vi "InitCamera.vi"(3 "error in":errorcluster, 5 "Scan.lvclass":refnum<class "Scan.lvclass">) -> (0 "error out":errorcluster, 2 "Initialized Camera":T2)   [LabVIEW 2017]
doc: "Creates, and edits acquisitions using the NI Vision Acquisition Express VI.\n\nThe NI Vision Acquisition Wizard is launched by placing the Express VI on the block diagram. Select an acquisition source and configure an acquisition using NI-IMAQ, NI-IMAQdx, or simulate an acquisition by reading an AVI or image files from a folder. After an acquisition is configured, select controls and indicators to be able to programmatically set in LabVIEW. Double-click the Vision Acquisition Express VI to edit the acquisition.\n\nNote: Any images created by the Express VI need to be disposed after use. Use the IMAQ Dispose.vi to cleanup the images output by the Express VI when they are no longer needed."
uses:
  classes/Scans/Scan.lvclass
  <vilib>/vision/Image Controls.llb/IMAQ Image.ctl
  classes/Scans/Scan.lvclass/Scan.ctl
  classes/Scans/Read A scans.vi
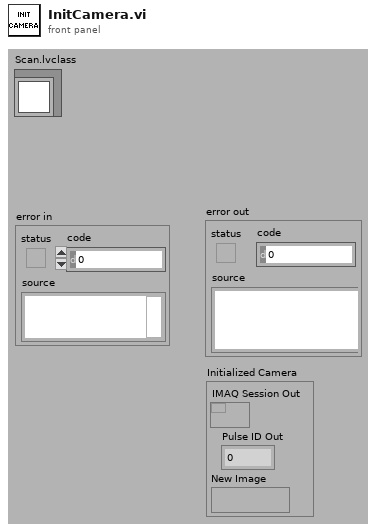
[diagram p1: front panel]
types:
  T1 = typedef "IMAQ Image.ctl" = refnum<image>
  T2 = cluster{"IMAQ Session Out":refnum<k11>, "Pulse ID Out":u32, "New Image":T1}
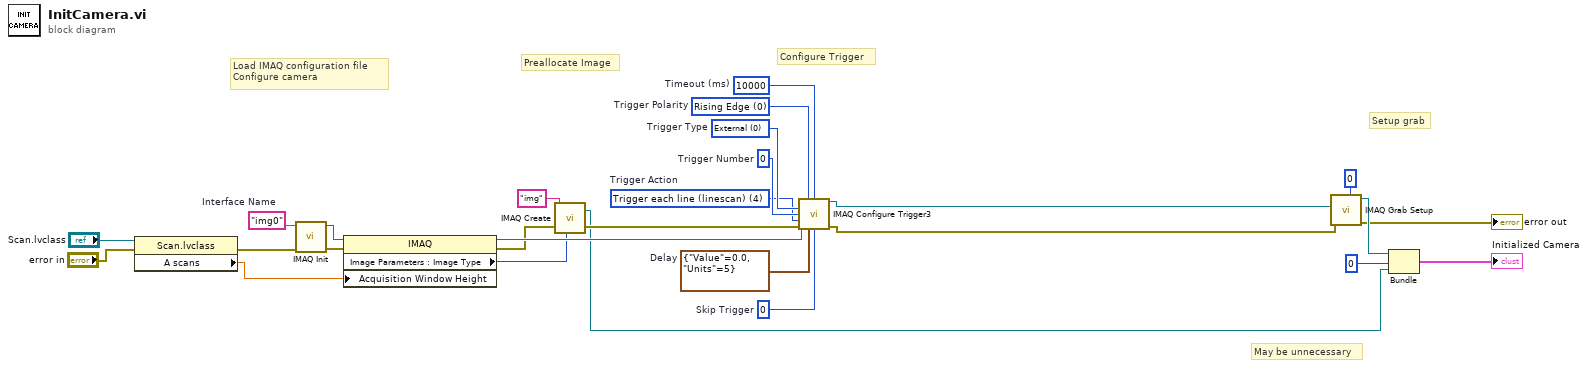
[diagram p0: block diagram]
diagram:
  w13 = cluster{"Value":dbl, "Units":u32} {"Value"=0.0, "Units"=5}  # Delay
  w16 = u32 10000  # Timeout (ms)
  w17 = u32 0 items=["Rising Edge", "Falling Edge"]  # Trigger Polarity
  w19 = u32 0  # Skip Trigger
  w14 = u32 4 items=["Disabled", "Trigger start of acquisition", "Trigger start of each buffer list", "Trigger each buffer", "Trigger each line (linescan)", "Trigger end of acquisition"]  # Trigger Action
  w15 = u32 0  # Trigger Number
  w18 = u32 0 items=["External"=0, "RTSI"=1, "ISO In"=2, "Scaled Encoder"=5]  # Trigger Type
  w20 = "img0"  # Interface Name
  # "May be unnecessary"
  # "Preallocate Image"
  # "Setup grab"
  # "Load IMAQ configuration file\nConfigure camera"
  # "Configure Trigger"
  n1 = property class="Scan.lvclass"(reference="Scan.lvclass", error in="error in") -> (error out=w9:errorcluster, "A scans"=w2:dbl)  [unwired: 1 out]
  n2 = call <vilib>:"IMAQ Init.vi"("error in (no error)"=w9, "Interface Name"=w20) -> ("error out"=w22:errorcluster, "IMAQ Session Out"=w4:refnum<k11>)  [unwired: 8 out]
  n3 = property class="IMAQ"(reference=w4, error in=w22, "Acquisition Window Height"=w2) -> (reference out=w27:refnum<k11>, error out=w21:errorcluster, "Image Parameters : Image Type"=w23:u32)
  n4 = call "IMAQ Create"("Image Name"="img", "Image Type"=w23, "error in (no error)"=w21) -> ("New Image"=w6:T1, "error out"=w26:errorcluster)  [unwired: 1 in, 1 out]
  n5 = call <vilib>:"IMAQ Configure Trigger3.vi"("IMAQ Session In"=w27, "Polarity"=w17, "Frame timeout (ms)"=w16, "Type"=w18, "Line Number"=w15, "Action"=w14, "error in (no error)"=w26, "Delay"=w13, "Skip trigger (linescan only)"=w19) -> ("IMAQ Session Out"=w24:refnum<k11>, "error out"=w25:errorcluster)  [unwired: 5 out]
  n6 = call <vilib>:"IMAQ Grab Setup.vi"("Channel"=0, "error in (no error)"=w25, "IMAQ Session In"=w24) -> ("error out"=→"error out":errorcluster, "IMAQ Session Out"=w8:refnum<k11>)  [unwired: 7 out]
  n7 = Bundle("IMAQ Session Out"=w8, "Pulse ID Out"=u32 0, "New Image"=w6) -> (→"Initialized Camera":T2)  [unwired: 1 in]
